vi "StarTrekIndicator.vi"() -> (1 "out":bool[](array[boolean]))   [LabVIEW 2019, in "Instrument.OxfordVRM UI.lvclass"]
uses:
  Instrument.OxfordVRM UI.lvclass
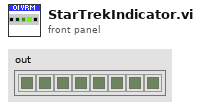
[diagram p1: front panel]
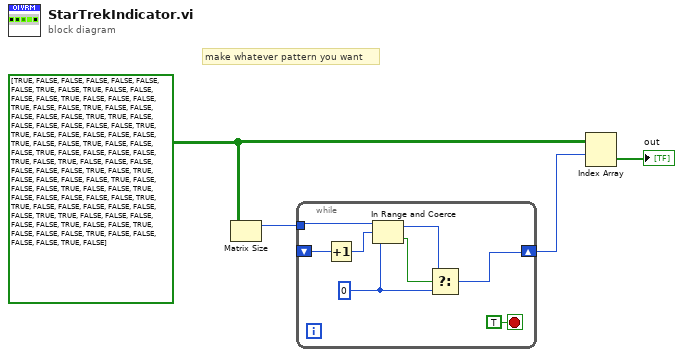
[diagram p0: block diagram]
diagram:
  w2 = bool[][] [[TRUE, FALSE, FALSE, FALSE, FALSE, FALSE, FALSE, TRUE], [FALSE, TRUE, FALSE, FALSE, FALSE, FALSE, TRUE, FALSE], [FALSE, FALSE, TRUE, FALSE, FALSE, TRUE, FALSE, FALSE], [FALSE, FALSE, FALSE, TRUE, TRUE, FALSE, FALSE, FALSE], [FALSE, FALSE, FALSE, TRUE, TRUE, FALSE, FALSE, FALSE], [FALSE, FALSE, TRUE, FALSE, FALSE, TRUE, FALSE, FALSE], [FALSE, TRUE, FALSE, FALSE, FALSE, FALSE, TRUE, FALSE], [TRUE, FALSE, FALSE, FALSE, FALSE, FALSE, FALSE, TRUE], [FALSE, TRUE, FALSE, FALSE, FALSE, FALSE, TRUE, FALSE], [FALSE, FALSE, TRUE, FALSE, FALSE, TRUE, FALSE, FALSE], [FALSE, FALSE, FALSE, TRUE, TRUE, FALSE, FALSE, FALSE], [FALSE, FALSE, FALSE, TRUE, TRUE, FALSE, FALSE, FALSE], [FALSE, FALSE, TRUE, FALSE, FALSE, TRUE, FALSE, FALSE], [FALSE, TRUE, FALSE, FALSE, FALSE, FALSE, TRUE, FALSE]] ("out")
  # "make whatever pattern you want"
  n1 = Matrix Size(0:w2) -> (1:w1:i32)  [unwired: 1 out]
  n2 = while {
    shift-right: [w7] -> w3
    shift-left: _ -> [w10]
    tunnel: w1 -> [w11]
    stop <- TRUE stop-if-true
    w6 = 0
    n3 = Increment(x=w10) -> (x+1=w5:i32)
    n4 = In Range and Coerce(upper limit=w11, x=w5, lower limit=w6) -> (coerced(x)=w8:i32, In Range?=w9:bool)
    n5 = Select(t=w8, s=w9, f=w6) -> (s? t:f=w7:i32)
  }
  n6 = Index Array(array=w2, index (row)=w3) -> (element=→"out":bool[])  [unwired: 1 in]
